vi "AH Bridge Avg Times.vi"(0 "VISA Resource name":refnum<visa-resource-name>, 1 "Is model 2500?":bool) -> (4 "Min Setting":u32, 5 "Wait Time (mS)":u32, 6 "VISA Resource out":refnum<visa-resource-name>, 7 "Setting":u32(slide)=4 max=15 step=1, 8 "Averaging Time":string[](array[string])=["0.029", "0.038", "0.050", "0.073", "0.111", "0.166", "0.260", "0.984", "1.460", "2.240", "3.780", "6.400", "11.800", "22.400", "45.400", "92.000"], 9 "Frequency":dbl)   [LabVIEW 2020]
panel:
  # "Index"
  # "0"
  # "1"
  # "2"
  # "3"
  # "4"
  # "5"
  # "6"
  # "7"
  # "8"
  # "9"
  # "10"
  # "11"
  # "12"
  # "13"
  # "14"
  # "15"
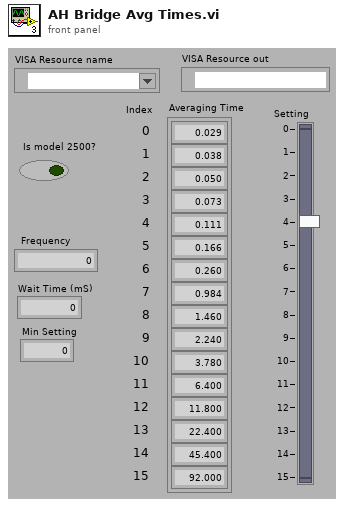
[diagram p1: front panel]
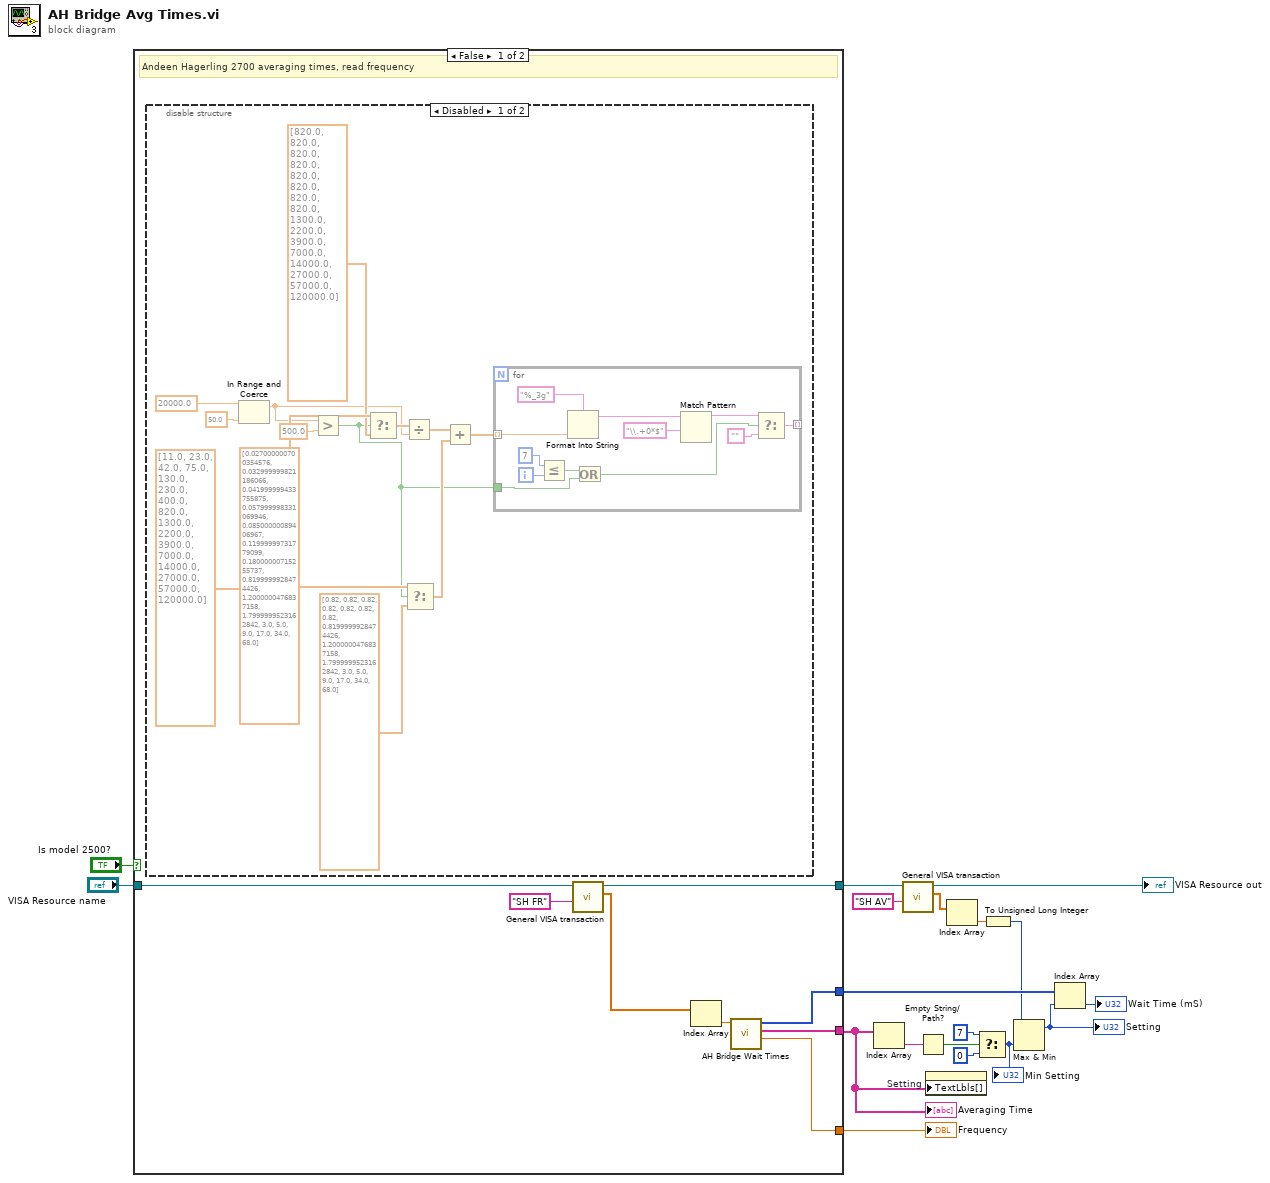
[diagram p0: block diagram]
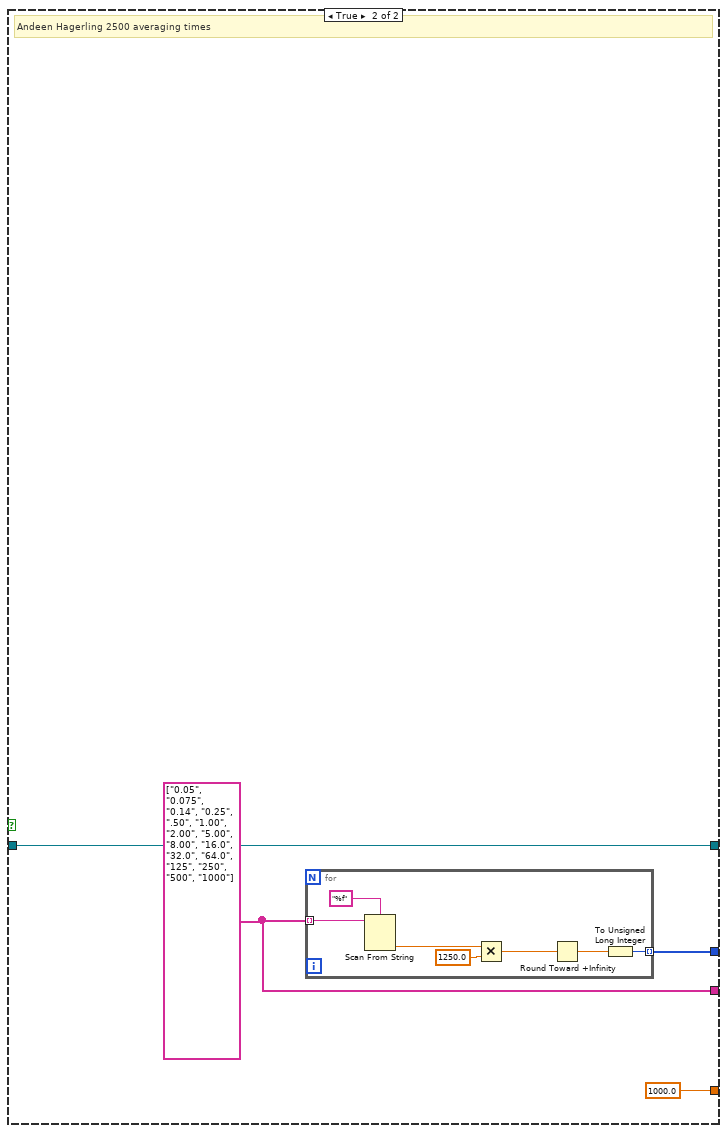
[diagram p3: hidden frame]
diagram:
  n1 = case shown="False" "Is model 2500?" {
    tunnel: [w21 1000.0 ("Frequency")] -> w17
    tunnel: "VISA Resource name" -> [w24 w52]
    tunnel: [w22 w54] -> w11
    tunnel: [w20 w53] -> w10
    tunnel: [w19 w52] -> w4
    frame False {
      # "Andeen Hagerling 2700 averaging times, read frequency"
      n2 = disable-structure shown="Disabled" {
        frame Disabled {
          n3 = In Range and Coerce(upper limit=20000.0, lower limit=50.0) -> (coerced(x)=w28:dbl)  [unwired: 1 in, 1 out]
          n4 = Greater?(x=w28, y=500.0) -> (0:w27:bool)
          n5 = Select(t=dbl[] [11.0, 23.0, 42.0, 75.0, 130.0, 230.0, 400.0, 820.0, 1300.0, 2200.0, 3900.0, 7000.0, 14000.0, 27000.0, 57000.0, 120000.0], s=w27, f=dbl[] [820.0, 820.0, 820.0, 820.0, 820.0, 820.0, 820.0, 820.0, 1300.0, 2200.0, 3900.0, 7000.0, 14000.0, 27000.0, 57000.0, 120000.0]) -> (s? t:f=w32:dbl[])
          n6 = Divide(x=w32, y=w28) -> (x/y=w38:dbl[])
          n7 = Select(t=dbl[] [0.027000000700354576, 0.032999999821186066, 0.041999999433755875, 0.057999998331069946, 0.08500000089406967, 0.11999999731779099, 0.18000000715255737, 0.8199999928474426, 1.2000000476837158, 1.7999999523162842, 3.0, 5.0, 9.0, 17.0, 34.0, 68.0], s=w27, f=dbl[] [0.82, 0.82, 0.82, 0.82, 0.82, 0.82, 0.82, 0.8199999928474426, 1.2000000476837158, 1.7999999523162842, 3.0, 5.0, 9.0, 17.0, 34.0, 68.0]) -> (s? t:f=w34:dbl[])
          n8 = Add(x=w38, y=w34) -> (x+y=w37:dbl[])
          n9 = for {
            tunnel: w37 -> [w51] mode=indexing
            tunnel: [w43] -> _ mode=indexing
            tunnel: w27 -> [w44]
            i -> [w47]
            n10 = Less Or Equal?(x=7, y=w47) -> (x <= y?=w45:bool)
            n11 = Format Into String(format string="%_3g", w51) -> (resulting string=w49:string)  [unwired: 2 in, 1 out]
            n12 = Or(x=w45, y=w44) -> (x .or. y?=w41:bool)
            n13 = Match Pattern(string=w49, regular expression="\\.+0*$") -> (before substring=w42:string)  [unwired: 1 in, 3 out]
            n14 = Select(t=w42, s=w41, f="") -> (s? t:f=w43:string)
          }
        }
        frame Enabled {
        }
      }
      n15 = call "General VISA transaction.vi"("Command String"="SH FR", "VISA Session"=w24) -> ("Measurement"=w26:dbl[], "dup VISA Session"=w19:refnum<visa-resource-name>)  [unwired: 4 in, 4 out]
      n16 = Index Array(array=w26) -> (element=w23:dbl)  [unwired: 1 in]
      n17 = call "AH Bridge Wait Times.vi"("Frequency"=w23) -> ("Frequency Out"=w21:dbl, "Averaging Time"=w22:string[], "Wait Time (mS)"=w20:u32[])  [unwired: 8 in]
    }
    frame True {
      w54 = string[] ["0.05", "0.075", "0.14", "0.25", ".50", "1.00", "2.00", "5.00", "8.00", "16.0", "32.0", "64.0", "125", "250", "500", "1000"] ("TextLbls[]")
      # "Andeen Hagerling 2500 averaging times"
      n18 = for {
        tunnel: w54 -> [w62] mode=indexing
        tunnel: [w56] -> w53 mode=indexing
        n19 = Scan From String(format string="%f", input string=w62) -> (output 1=w60:dbl)  [unwired: 3 in, 3 out]
        n20 = Multiply(x=w60, y=1250.0) -> (x*y=w58:dbl)
        n21 = Round Toward +Infinity(x=w58) -> (ceil(x): smallest int >= x=w57:dbl)
        n22 = To Unsigned Long Integer(number=w57) -> (unsigned 32bit integer=w56:u32)
      }
    }
  }
  "Averaging Time" <- w11
  "Frequency" <- w17
  n23 = Index Array(array=w11) -> (element=w16:string)  [unwired: 1 in]
  n24 = call "General VISA transaction.vi"("Command String"="SH AV", "VISA Session"=w4) -> ("Measurement"=w6:dbl[], "dup VISA Session"=→"VISA Resource out":refnum<visa-resource-name>)  [unwired: 4 in, 4 out]
  n25 = Empty String/Path?(string/path=w16) -> (empty?=w15:bool)
  n26 = property on="Setting" class="Slide (strict)"("TextLbls[]"=w11) -> ()  [unwired: 2 in, 2 out]
  n27 = Index Array(array=w6) -> (element=w7:dbl)  [unwired: 1 in]
  n28 = Select(t=u32 7 ("unsigned 32bit integer"), s=w15, f=u32 0) -> (s? t:f=w12:u32)
  "Min Setting" <- w12
  n29 = To Unsigned Long Integer(number=w7) -> (unsigned 32bit integer=w2:u32)
  n30 = Max & Min(x=w2, y=w12) -> (max(x,y)=w9:u32)  [unwired: 1 out]
  "Setting" <- w9
  n31 = Index Array(array=w10, index=w9) -> (element=→"Wait Time (mS)":u32)
